vi "Check Delay Dependencies.vi"(7 "Problem Chnls in":string[](array[string]), 8 "error in (no error)":errorcluster, 9 "new Delay":dbl, 10 "Chnl":string, 11 "BME_DG_System in":refnum<class "BME_DG_System.lvclass">) -> (0 "error out":errorcluster, 2 "Dependecies OK":bool, 3 "BME_DG_System out":refnum<class "BME_DG_System.lvclass">, 5 "Problem Chnls out":string[](array[string]))   [LabVIEW 2009, in "BME_DG_System.lvclass"]
uses:
  BME_DG_System.lvclass
  BME_DG_System.lvclass/BME_DG_System.ctl
  BME_DG_Base/BME_DG_Base.lvclass
  BME_DG_Chnl/BME_DG_Chnl.lvclass
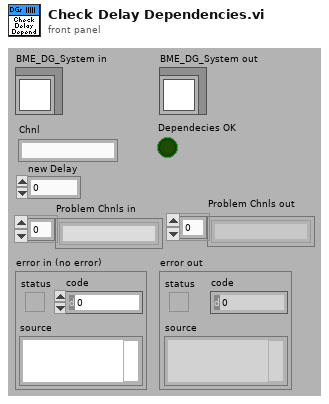
[diagram p1: front panel]
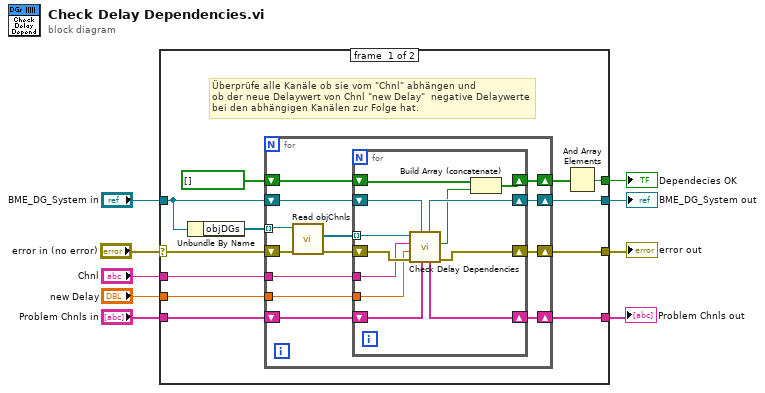
[diagram p0: block diagram]
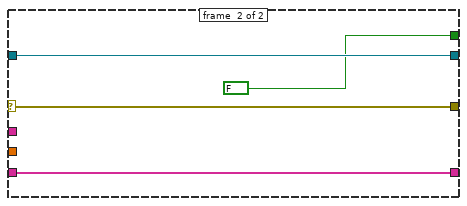
[diagram p2: hidden frame]
diagram:
  n1 = case shown="No Error" "error in (no error)" {
    selector: "error in (no error)" -> [w19 w50]
    tunnel: [w15 w50] -> w8
    tunnel: [w18 w49] -> w6
    tunnel: "BME_DG_System in" -> [w20 w49]
    tunnel: "Chnl" -> [w17 _]
    tunnel: "new Delay" -> [w16 _]
    tunnel: [w14 FALSE] -> w3
    tunnel: "Problem Chnls in" -> [w13 w47]
    tunnel: [w12 w47] -> w1
    frame #0 {
      # "Überprüfe alle Kanäle ob sie vom \"Chnl\" abhängen und \nob der neue Delaywert von Chnl \"new Delay\"  negative Delaywerte\nbei den abhängigen Kanälen zur Folge hat."
      n2 = Unbundle By Name(w20) -> ("objDGs"=w21:refnum<class "BME_DG_Base.lvclass">[])
      n3 = for {
        tunnel: w21 -> [w34] mode=indexing
        shift-right: [w29] -> w18
        shift-left: w20 -> [w32]
        shift-right: [w28] -> w15
        shift-left: w19 -> [w31]
        tunnel: w17 -> [w27]
        tunnel: w16 -> [w26]
        shift-right: [w24] -> w12
        shift-left: w13 -> [w25]
        shift-right: [w22] -> w10
        shift-left: bool[] [] -> [w23]
        n4 = call-dynamic "Read objChnls.vi"("error in (no error)"=w31, "BME_DG_Base in"=w34) -> ("error out"=w30:errorcluster, "objChnls"=w33:refnum<class "BME_DG_Chnl.lvclass">[])  [unwired: 6 in, 2 out]
        n5 = for {
          tunnel: w33 -> [w46] mode=indexing
          shift-right: [w42] -> w29
          shift-left: w32 -> [w43]
          shift-right: [w44] -> w28
          shift-left: w30 -> [w45]
          tunnel: w27 -> [w41]
          tunnel: w26 -> [w40]
          shift-right: [w38] -> w24
          shift-left: w25 -> [w39]
          shift-right: [w36] -> w22
          shift-left: w23 -> [w37]
          n6 = call "Check Delay Dependencies.vi"("Problem Chnls in"=w39, "BME_DG_System"=w43, "error in (no error)"=w45, "new Delay"=w40, "Chnl"=w41, "BME_DG_Chnl in"=w46) -> ("error out"=w44:errorcluster, "Dependecies OK"=w35:bool, "Problem Chnls out"=w38:string[], "BME_DG_System out"=w42:refnum<class "BME_DG_System.lvclass">)  [unwired: 1 in, 1 out]
          n7 = Build Array (concatenate)(w37, w35) -> (w36:bool[])
        }
      }
      n8 = And Array Elements(Boolean array=w10) -> (logical AND=w14:bool)
    }
    frame #1 {
    }
  }
  "error out" <- w8
  "BME_DG_System out" <- w6
  "Dependecies OK" <- w3
  "Problem Chnls out" <- w1
